vi "Obtain Request Events.vi"(8 "error in (no error)":errorcluster, 10 "Create New?":bool) -> (0 "error out":errorcluster, 2 "Tool Module Request Events":T1)   [LabVIEW 2015, in "Tool Module.lvlib"]
doc: "This VI Obtains/Creates the Requests events that will be used for other modules to communicate with the module that owns this VI. These Requests events will be accessed only via Public API methods for this module.\n\n<b>NOTE</b>: The contents of this VI are automatically generated and modified by the <b>Tools > Delacor > DQMH</b> utilities. Consider using those utilities instead of making your own modifications to this VI.\n_____\nBased on Delacor QMH Project Template 2.1.0.2."
uses:
  Tool Module.lvlib
  Request Events--cluster.ctl
  Stop Argument--cluster.ctl
  Get Module Execution Status Argument--cluster.ctl
  Show Diagram Argument--cluster.ctl
  Test Trig 2 Argument--cluster.ctl
  Support/Timer Setup Params Typedef.ctl
  GOTO Argument--cluster.ctl
  Support/_GoTo Cmd Typedef--enum.ctl
  Start Inspect Argument--cluster.ctl
  Support/_Sample Data Rtn Cluster--typedef.ctl
  CONNECT Argument--cluster.ctl
  Get All Inspect Data Argument--cluster.ctl
  Get All Inspect Data (Reply Payload)--cluster.ctl
  Get Inspection Limits Argument--cluster.ctl
  Get Inspection Limits (Reply Payload)--cluster.ctl
  Set Inspection Limits Argument--cluster.ctl
  Support/_Inspection Limits cluster--typedef.ctl
  Update Status Argument--cluster.ctl
  Start Data Monitor Argument--cluster.ctl
  Get FPGA Setup Params Argument--cluster.ctl
  Get FPGA Setup Params (Reply Payload)--cluster.ctl
  Tool Typedefs/_FPGA Setup Params Cluster--typedef.ctl
  Tool Typedefs/_FPGA Timing Constraints Cluster--typedef.ctl
  Tool Typedefs/_FPGA Timing Ctrl Cluster--typedef.ctl
  Tool Typedefs/_FPGA Laser Config Cluster--typedef.ctl
  Tool Typedefs/_FPGA Peak Proc Cfg Cluster--typedef.ctl
  Tool Typedefs/_FPGA SPI Cfg Cluster--typedef.ctl
  Set FPGA Setup Params Argument--cluster.ctl
  Set Tool Config Argument--cluster.ctl
  Tool Config/_Configuration Cluster_v3--typedef.ctl
  Tool Config/_Tool Block Cluster_v3--typedef.ctl
  Tool Config/_Motor Block Cluster_v2--typedef.ctl
  Tool Config/_Verification Blk Cluster--typedef.ctl
  Tool Config/_ProbeConfigParams Cluster--typedef.ctl
  Tool Config/_Sensor Block Cluster--typedef.ctl
  Tool Config/_SensorConfigParams Cluster--typedef.ctl
  Get Tool Config Argument--cluster.ctl
  Get Tool Config (Reply Payload)--cluster.ctl
  Set Integration Count Argument--cluster.ctl
  Set Laser Params Argument--cluster.ctl
  Get Mtrl Ctrl Reg Argument--cluster.ctl
  Get Mtrl Ctrl Reg (Reply Payload)--cluster.ctl
  Commit Ctrl Reg Argument--cluster.ctl
  Set Event Logger Argument--cluster.ctl
  Event Logger Library/Event Log/EventLog.lvclass
  Write to File Argument--cluster.ctl
  Read from File Argument--cluster.ctl
  Set Device Temp Thresholds Argument--cluster.ctl
  Tool Typedefs/_Temperature Threshold Arrays--typedef.ctl
  Get Cycle Count Argument--cluster.ctl
  Get Cycle Count (Reply Payload)--cluster.ctl
  Return FPGA Setup Data Argument--cluster.ctl
  Return FPGA Setup Data (Reply Payload)--cluster.ctl
  Update FPGA Setup Data Argument--cluster.ctl
  Tool Config/Tool Cfg.lvlib
panel:
  # "NOTE: The contents of this VI are automatically generated and modified by the Tools > Delacor > DQMH utilities. Consider using those utilities instead of making your own modifications to this VI."
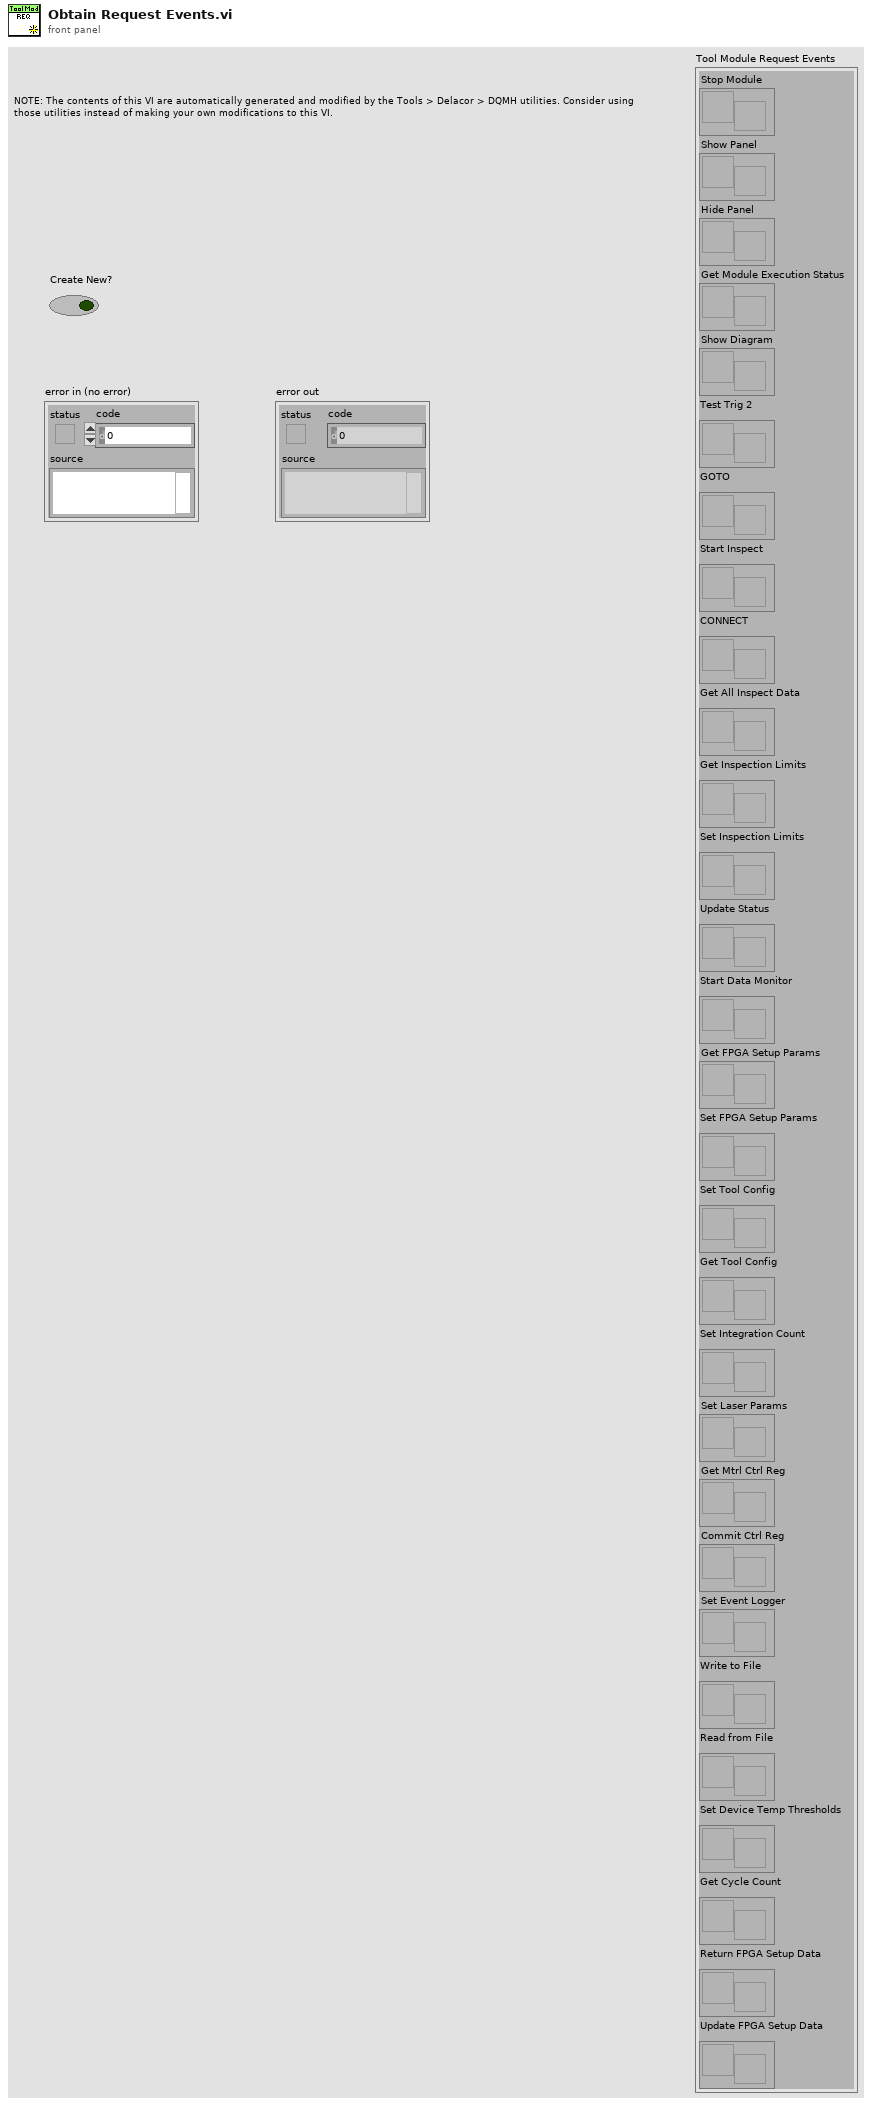
[diagram p1: front panel]
types:
  T1 = typedef "Tool Module.lvlib/Request Events--cluster.ctl" = cluster{"Stop Module":refnum<user-event>, "Show Panel":refnum<user-event>, "Hide Panel":refnum<user-event>, "Get Module Execution Status":refnum<user-event>, "Show Diagram":refnum<user-event>, "Test Trig 2":refnum<user-event>, "GOTO":refnum<user-event>, "Start Inspect":refnum<user-event>, "CONNECT":refnum<user-event>, "Get All Inspect Data":refnum<user-event>, "Get Inspection Limits":refnum<user-event>, "Set Inspection Limits":refnum<user-event>, "Update Status":refnum<user-event>, "Start Data Monitor":refnum<user-event>, "Get FPGA Setup Params":refnum<user-event>, "Set FPGA Setup Params":refnum<user-event>, "Set Tool Config":refnum<user-event>, "Get Tool Config":refnum<user-event>, "Set Integration Count":refnum<user-event>, "Set Laser Params":refnum<user-event>, "Get Mtrl Ctrl Reg":refnum<user-event>, "Commit Ctrl Reg":refnum<user-event>, "Set Event Logger":refnum<user-event>, "Write to File":refnum<user-event>, "Read from File":refnum<user-event>, "Set Device Temp Thresholds":refnum<user-event>, "Get Cycle Count":refnum<user-event>, "Return FPGA Setup Data":refnum<user-event>, "Update FPGA Setup Data":refnum<user-event>}
  T2 = typedef "Tool Module.lvlib/Update FPGA Setup Data Argument--cluster.ctl" = cluster{"Commit":bool, "FPGA Setup Parameters":T3}
  T3 = typedef "_FPGA Setup Params Cluster--typedef.ctl" = cluster{"FPGA Timing Constraints":T4, "FPGA Timing Ctrl":T5, "FPGA Laser Config":T6, "FPGA Peak Proc Cfg":T7, "FPGA SPI Cfg":T8}
  T4 = typedef "_FPGA Timing Constraints Cluster--typedef.ctl" = cluster{"frame.length Min":u16, "frame.ST_OFF Min":u16, "frame.ST_ON Min":u16, "frame.first data idx":u16, "frame.integ Offset":u16, "frame.integ Delay":u16, "frame.ad_latch Delay":u16, "frame.trig time Max":u32}
  T5 = typedef "_FPGA Timing Ctrl Cluster--typedef.ctl" = cluster{"trig.time":u32, "integ.count 1":u32, "integ.count 2":u32, "encdr.latch ctrl":u32, "pixel.read count":u16, "clock.select":u16, "ad.clock offset":u16, "data.control reg":u16}
  T6 = typedef "_FPGA Laser Config Cluster--typedef.ctl" = cluster{"laser.gain":i16, "laser.threshold Low":u16, "laser.threshold High":u16, "laser.dac init":u16, "laser.dac Min":u16, "laser.dac Max":u16, "laser.config reg":u16}
  T7 = typedef "_FPGA Peak Proc Cfg Cluster--typedef.ctl" = cluster{"PD.threshold":u16, "PD.width detect Min":u8, "PD.sensor pixels":u16, "PD.config reg":u16}
  T8 = typedef "_FPGA SPI Cfg Cluster--typedef.ctl" = cluster{"SPI Divide Value":u8, "SPI config reg":u16}
  T9 = typedef "Tool Module.lvlib/Return FPGA Setup Data Argument--cluster.ctl" = cluster{"Reload":bool, "Wait Notifier":refnum<notifier>, "wait for reply":bool}
  T10 = typedef "Tool Module.lvlib/Get Cycle Count Argument--cluster.ctl" = cluster{"Clear?":bool, "Wait Notifier":refnum<notifier>}
  T11 = typedef "Tool Module.lvlib/Set Device Temp Thresholds Argument--cluster.ctl" = cluster{"Device Temp Thold Arrays":T12}
  T12 = typedef "_Temperature Threshold Arrays--typedef.ctl" = cluster{"High Thold ":dbl[], "Low Thold ":dbl[]}
  T13 = typedef "Tool Module.lvlib/Read from File Argument--cluster.ctl" = cluster{"Filename":string, "Create?":bool, "Flattened Data Strings":string[]}
  T14 = typedef "Tool Module.lvlib/Write to File Argument--cluster.ctl" = cluster{"Filename":string, "Flattened data strings":string[]}
  T15 = typedef "Tool Module.lvlib/Set Event Logger Argument--cluster.ctl" = cluster{"EventLog.lvclass":refnum<class "EventLog.lvclass">}
  T16 = typedef "Tool Module.lvlib/Commit Ctrl Reg Argument--cluster.ctl" = cluster{"Ctrl Reg":u16}
  T17 = typedef "Tool Module.lvlib/Get Mtrl Ctrl Reg Argument--cluster.ctl" = cluster{"dummy":bool, "Wait Notifier":refnum<notifier>}
  T18 = typedef "Tool Module.lvlib/Set Laser Params Argument--cluster.ctl" = cluster{"Mode":i16, "Gain":u16, "Init DAC":u16}
  T19 = typedef "Tool Module.lvlib/Set Integration Count Argument--cluster.ctl" = cluster{"Mode":i16, "Integ Count":u32}
  T20 = typedef "Tool Module.lvlib/Get Tool Config Argument--cluster.ctl" = cluster{"dummy":bool, "Wait Notifier":refnum<notifier>}
  T21 = typedef "Tool Module.lvlib/Set Tool Config Argument--cluster.ctl" = cluster{"Commit":bool, "Tool Config Cluster":T22}
  T22 = typedef "Tool Cfg.lvlib/_Configuration Cluster_v3--typedef.ctl" = cluster{"Tool Type":u16, "Tool SN":u16, "Tool Block":T23, "Motor Block":T24, "Verification Block":T25, "Probe Block":cluster{"nProbes":u16, "Probe Param Array":T26[]}}
  T23 = typedef "Tool Cfg.lvlib/_Tool Block Cluster_v3--typedef.ctl" = cluster{"Encoder Size":u16, "Encoder Scale":u32, "Encoder Offset":i32, "MaxEncoder":i32, "MinEncoder":i32, "Start Delay":sgl, "Tool Face Ref":sgl}
  T24 = typedef "Tool Cfg.lvlib/_Motor Block Cluster_v2--typedef.ctl" = cluster{"MinMotor Speed":u16, "MaxMotor Speed":u16, "Homing Speed":u16, "Jog Speed":u16, "Inspect Speed":u16, "VBlk Speed":u16, "CleaningPos":i32, "Safe Zone":i32, "Has Motor":bool, "Use Home Index":bool}
  T25 = typedef "Tool Cfg.lvlib/_Verification Blk Cluster--typedef.ctl" = cluster{"Angle":sgl, "FlankLength1":sgl, "FlankLength2":sgl, "Location":sgl, "Serial Number":u16}
  T26 = typedef "Tool Cfg.lvlib/_ProbeConfigParams Cluster--typedef.ctl" = cluster{"Name":string, "Laser Init Pwr":u16, "Laser Gain":u8, "Integ Count":u16, "Meas. Range":sgl, "Angle":sgl, "Probe Offset":sgl, "Sensor Block":T27}
  T27 = typedef "Tool Cfg.lvlib/_Sensor Block Cluster--typedef.ctl" = cluster{"nSensors":u16, "SensorCfgParams Array":T28[]}
  T28 = typedef "Tool Cfg.lvlib/_SensorConfigParams Cluster--typedef.ctl" = cluster{"Total Pixels":u16, "Positive  Peaks":bool, "CalibrCoefArray":dbl[], "Start Idx":u16, "End Idx":u16}
  T29 = typedef "Tool Module.lvlib/Set FPGA Setup Params Argument--cluster.ctl" = cluster{"Commit":bool, "FPGA Setup Parameters":T3}
  T30 = typedef "Tool Module.lvlib/Get FPGA Setup Params Argument--cluster.ctl" = cluster{"dummy":bool, "Wait Notifier":refnum<notifier>}
  T31 = typedef "Tool Module.lvlib/Start Data Monitor Argument--cluster.ctl" = cluster{"Monitor":bool, "Lasers ON?":bool, "Host Sample Data notifier":refnum<notifier>}
  T32 = typedef "Tool Module.lvlib/Update Status Argument--cluster.ctl" = cluster{"Encoder":i32, "STATUS":u16, "MC SM State":u16, "M_Ctrl":u16}
  T33 = typedef "Tool Module.lvlib/Set Inspection Limits Argument--cluster.ctl" = cluster{"Inspection Limits":T34}
  T34 = typedef "Tool Module.lvlib/_Inspection Limits cluster--typedef.ctl" = cluster{"MaxSamples":i32, "PosToStartScan":i32, "PosToEndScan":i32, "ScanLength":i32}
  T35 = typedef "Tool Module.lvlib/Get Inspection Limits Argument--cluster.ctl" = cluster{"dummy":bool, "Wait Notifier":refnum<notifier>}
  T36 = typedef "Tool Module.lvlib/Get All Inspect Data Argument--cluster.ctl" = cluster{"dummy":bool, "Wait Notifier":refnum<notifier>}
  T37 = typedef "Tool Module.lvlib/CONNECT Argument--cluster.ctl" = cluster{"Connect":bool}
  T38 = typedef "Tool Module.lvlib/Start Inspect Argument--cluster.ctl" = cluster{"Inspect":bool, "Host Sample Data notifier":refnum<notifier>}
  T39 = typedef "Tool Module.lvlib/GOTO Argument--cluster.ctl" = cluster{"GoTo Cmd":T40, "Data":i32}
  T40 = typedef "Tool Module.lvlib/_GoTo Cmd Typedef--enum.ctl" = enum16{"MoveA", "MoveR", "Home Position", "Home None", "Cleaning Position"}
  T41 = typedef "Tool Module.lvlib/Test Trig 2 Argument--cluster.ctl" = cluster{"Trigger Params":T42}
  T42 = typedef "Tool Module.lvlib/Timer Setup Params Typedef.ctl" = cluster{"Timer On":bool, "Period":i32, "Count":i32}
  T43 = typedef "Tool Module.lvlib/Show Diagram Argument--cluster.ctl" = cluster{"Debug?":bool}
  T44 = typedef "Tool Module.lvlib/Get Module Execution Status Argument--cluster.ctl" = cluster{"Running?":bool}
  T45 = typedef "Tool Module.lvlib/Stop Argument--cluster.ctl" = cluster{"Origin":string, "Exit via Stop Module Req?":bool, "Wait for Module to stop?":bool}
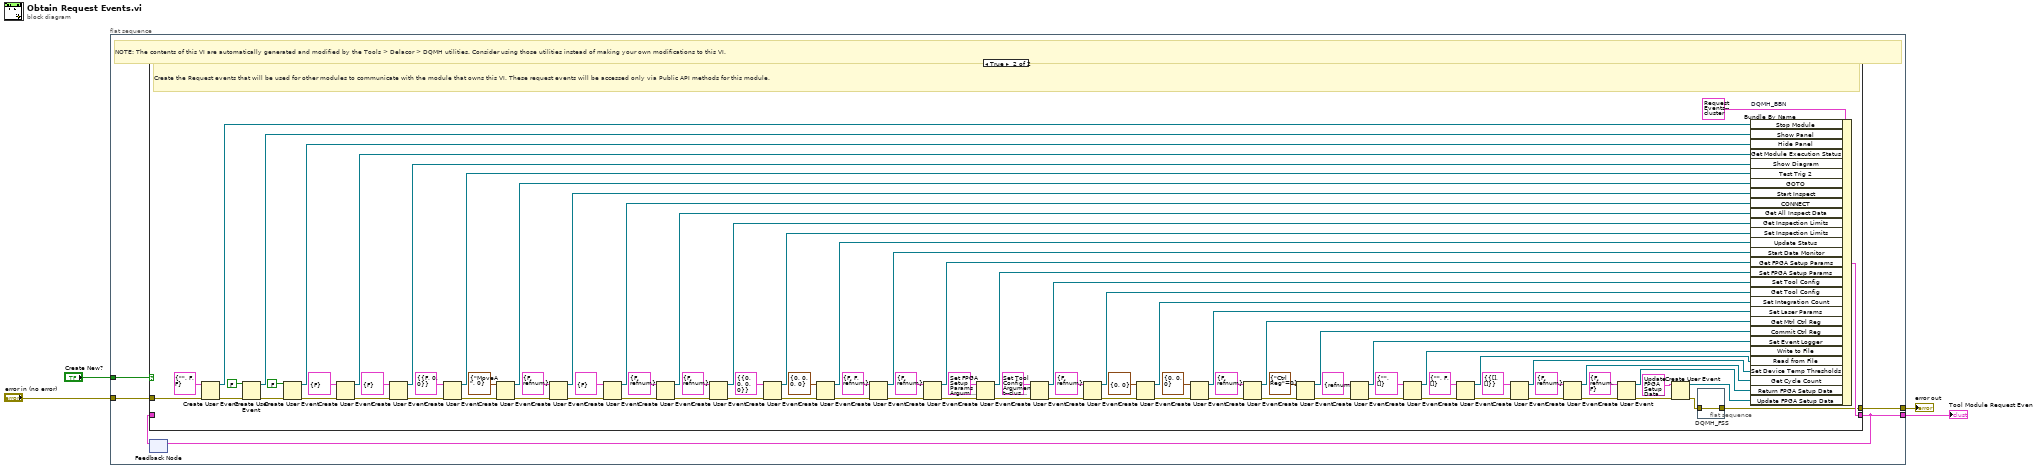
[diagram p0: block diagram]
diagram:
  n1 = flat-sequence {
    tunnel: [w9] -> w4
    tunnel: "error in (no error)" -> [w8]
    tunnel: [w6] -> w2
    tunnel: "Create New?" -> [w5]
    frame #0 {
      # "NOTE: The contents of this VI are automatically generated and modified by the Tools > Delacor > DQMH utilities. Consider using those utilities instead of making your own modifications to this VI."
      n2 = feedback #1() -> (w7:T1)  [unwired: 1 in]
      n3 = case shown="True" w5 {
        tunnel: [w10 w90] -> w9
        tunnel: w8 -> [w10 w102]
        tunnel: [w11 w99] -> w6
        tunnel: w7 -> [w11 _]
        frame False {
          # "Obtain the Request events that were created in a previous call to this VI."
        }
        frame True {
          # "Create the Request events that will be used for other modules to communicate with the module that owns this VI. These request events will be accessed only via Public API methods for this module."
          n4 = Create User Event(user event datatype=T45 {"Origin"="", "Exit via Stop Module Req?"=FALSE, "Wait for Module to stop?"=FALSE} ("Stop Argument"), error in=w102) -> (user event=w100:refnum<user-event>, error out=w97:errorcluster)
          n5 = Create User Event(user event datatype=FALSE ("Show Panel"), error in=w97) -> (user event=w95:refnum<user-event>, error out=w93:errorcluster)
          n6 = Create User Event(user event datatype=FALSE ("Hide Panel"), error in=w93) -> (user event=w92:refnum<user-event>, error out=w91:errorcluster)
          n7 = Create User Event(user event datatype=T44 {"Running?"=FALSE} ("Get Module Execution Status Argument"), error in=w91) -> (user event=w88:refnum<user-event>, error out=w89:errorcluster)
          n8 = Create User Event(user event datatype=T43 {"Debug?"=FALSE} ("Show Diagram Argument"), error in=w89) -> (user event=w85:refnum<user-event>, error out=w86:errorcluster)
          n9 = Create User Event(user event datatype=T41 {"Trigger Params"={"Timer On"=FALSE, "Period"=0, "Count"=0}} ("Test Trig 2 Argument"), error in=w86) -> (user event=w82:refnum<user-event>, error out=w83:errorcluster)
          n10 = Create User Event(user event datatype=T39 {"GoTo Cmd"=enum."MoveA", "Data"=0} ("GOTO Argument"), error in=w83) -> (user event=w79:refnum<user-event>, error out=w80:errorcluster)
          n11 = Create User Event(user event datatype=T38 {"Inspect"=FALSE, "Host Sample Data notifier"=refnum} ("Start Inspect Argument"), error in=w80) -> (user event=w76:refnum<user-event>, error out=w77:errorcluster)
          n12 = Create User Event(user event datatype=T37 {"Connect"=FALSE} ("CONNECT Argument"), error in=w77) -> (user event=w73:refnum<user-event>, error out=w74:errorcluster)
          n13 = Create User Event(user event datatype=T36 {"dummy"=FALSE, "Wait Notifier"=refnum} ("Get All Inspect Data Argument"), error in=w74) -> (user event=w70:refnum<user-event>, error out=w71:errorcluster)
          n14 = Create User Event(user event datatype=T35 {"dummy"=FALSE, "Wait Notifier"=refnum} ("Get Inspection Limits Argument"), error in=w71) -> (user event=w67:refnum<user-event>, error out=w68:errorcluster)
          n15 = Create User Event(user event datatype=T33 {"Inspection Limits"={"MaxSamples"=0, "PosToStartScan"=0, "PosToEndScan"=0, "ScanLength"=0}} ("Set Inspection Limits Argument"), error in=w68) -> (user event=w64:refnum<user-event>, error out=w65:errorcluster)
          n16 = Create User Event(user event datatype=T32 {"Encoder"=0, "STATUS"=0, "MC SM State"=0, "M_Ctrl"=0} ("Update Status Argument"), error in=w65) -> (user event=w61:refnum<user-event>, error out=w62:errorcluster)
          n17 = Create User Event(user event datatype=T31 {"Monitor"=FALSE, "Lasers ON?"=FALSE, "Host Sample Data notifier"=refnum} ("Start Data Monitor Argument"), error in=w62) -> (user event=w58:refnum<user-event>, error out=w59:errorcluster)
          n18 = Create User Event(user event datatype=T30 {"dummy"=FALSE, "Wait Notifier"=refnum} ("Get FPGA Setup Params Argument"), error in=w59) -> (user event=w55:refnum<user-event>, error out=w56:errorcluster)
          n19 = Create User Event(user event datatype=T29 {"Commit"=FALSE, "FPGA Setup Parameters"={"FPGA Timing Constraints"={"frame.length Min"=530, "frame.ST_OFF Min"=15, "frame.ST_ON Min"=8, "frame.first data idx"=14, "frame.integ Offset"=6, "frame.integ Delay"=3, "frame.ad_latch Delay"=11, "frame.trig time Max"=0}, "FPGA Timing Ctrl"={"trig.time"=220, "integ.count 1"=400, "integ.count 2"=350, "encdr.latch ctrl"=1, "pixel.read count"=512, "clock.select"=2, "ad.clock offset"=16, "data.control reg"=2}, "FPGA Laser Config"={"laser.gain"=10, "laser.threshold Low"=1400, "laser.threshold High"=1900, "laser.dac init"=912, "laser.dac Min"=800, "laser.dac Max"=4000, "laser.config reg"=3}, "FPGA Peak Proc Cfg"={"PD.threshold"=0, "PD.width detect Min"=0, "PD.sensor pixels"=512, "PD.config reg"=23}, "FPGA SPI Cfg"={"SPI Divide Value"=1, "SPI config reg"=1}}} ("Set Cur FPGA Setup Params Argument"), error in=w56) -> (user event=w52:refnum<user-event>, error out=w53:errorcluster)
          n20 = Create User Event(user event datatype=T21 {"Commit"=FALSE, "Tool Config Cluster"={"Tool Type"=0, "Tool SN"=0, "Tool Block"={"Encoder Size"=0, "Encoder Scale"=0, "Encoder Offset"=0, "MaxEncoder"=0, "MinEncoder"=0, "Start Delay"=0.0, "Tool Face Ref"=0.0}, "Motor Block"={"MinMotor Speed"=0, "MaxMotor Speed"=0, "Homing Speed"=90, "Jog Speed"=90, "Inspect Speed"=90, "VBlk Speed"=90, "CleaningPos"=0, "Safe Zone"=0, "Has Motor"=FALSE, "Use Home Index"=FALSE}, "Verification Block"={"Angle"=90.0, "FlankLength1"=0.0, "FlankLength2"=0.0, "Location"=0.0, "Serial Number"=0}, "Probe Block"={"nProbes"=0, "Probe Param Array"=[]}}} ("Set Tool Config Argument"), error in=w53) -> (user event=w49:refnum<user-event>, error out=w50:errorcluster)
          n21 = Create User Event(user event datatype=T20 {"dummy"=FALSE, "Wait Notifier"=refnum} ("Get Tool Config Argument"), error in=w50) -> (user event=w46:refnum<user-event>, error out=w47:errorcluster)
          n22 = Create User Event(user event datatype=T19 {"Mode"=0, "Integ Count"=0} ("Set Integration Count Argument"), error in=w47) -> (user event=w43:refnum<user-event>, error out=w44:errorcluster)
          n23 = Create User Event(user event datatype=T18 {"Mode"=0, "Gain"=0, "Init DAC"=0} ("Set Laser Params Argument"), error in=w44) -> (user event=w40:refnum<user-event>, error out=w41:errorcluster)
          n24 = Create User Event(user event datatype=T17 {"dummy"=FALSE, "Wait Notifier"=refnum} ("Get Mtrl Ctrl Reg Argument"), error in=w41) -> (user event=w37:refnum<user-event>, error out=w38:errorcluster)
          n25 = Create User Event(user event datatype=T16 {"Ctrl Reg"=0} ("Set Mtr Ctrl Reg Argument"), error in=w38) -> (user event=w34:refnum<user-event>, error out=w35:errorcluster)
          n26 = Create User Event(user event datatype=T15 {"EventLog.lvclass"=refnum} ("Set Event Logger Argument"), error in=w35) -> (user event=w31:refnum<user-event>, error out=w32:errorcluster)
          n27 = Create User Event(user event datatype=T14 {"Filename"="", "Flattened data strings"=[]} ("Write to File Argument"), error in=w32) -> (user event=w28:refnum<user-event>, error out=w29:errorcluster)
          n28 = Create User Event(user event datatype=T13 {"Filename"="", "Create?"=FALSE, "Flattened Data Strings"=[]} ("Read from File Argument"), error in=w29) -> (user event=w25:refnum<user-event>, error out=w26:errorcluster)
          n29 = Create User Event(user event datatype=T11 {"Device Temp Thold Arrays"={"High Thold "=[], "Low Thold "=[]}} ("Set Device Temp Thresholds Argument"), error in=w26) -> (user event=w22:refnum<user-event>, error out=w23:errorcluster)
          n30 = Create User Event(user event datatype=T10 {"Clear?"=FALSE, "Wait Notifier"=refnum} ("Get Cycle Count Argument"), error in=w23) -> (user event=w19:refnum<user-event>, error out=w20:errorcluster)
          n31 = Create User Event(user event datatype=T9 {"Reload"=FALSE, "Wait Notifier"=refnum, "wait for reply"=FALSE} ("Return FPGA Setup Data Argument"), error in=w20) -> (user event=w16:refnum<user-event>, error out=w17:errorcluster)
          n32 = Create User Event(user event datatype=T2 {"Commit"=FALSE, "FPGA Setup Parameters"={"FPGA Timing Constraints"={"frame.length Min"=530, "frame.ST_OFF Min"=15, "frame.ST_ON Min"=8, "frame.first data idx"=14, "frame.integ Offset"=6, "frame.integ Delay"=3, "frame.ad_latch Delay"=11, "frame.trig time Max"=0}, "FPGA Timing Ctrl"={"trig.time"=220, "integ.count 1"=400, "integ.count 2"=350, "encdr.latch ctrl"=1, "pixel.read count"=512, "clock.select"=2, "ad.clock offset"=16, "data.control reg"=2}, "FPGA Laser Config"={"laser.gain"=10, "laser.threshold Low"=1400, "laser.threshold High"=1900, "laser.dac init"=912, "laser.dac Min"=800, "laser.dac Max"=4000, "laser.config reg"=3}, "FPGA Peak Proc Cfg"={"PD.threshold"=0, "PD.width detect Min"=0, "PD.sensor pixels"=512, "PD.config reg"=23}, "FPGA SPI Cfg"={"SPI Divide Value"=1, "SPI config reg"=1}}} ("Update FPGA Setup Data Argument"), error in=w17) -> (user event=w13:refnum<user-event>, error out=w14:errorcluster)
          n33 = flat-sequence "DQMH_FSS" {
            tunnel: w14 -> [w103]
            tunnel: [w103] -> w90
            frame #0 {
            }
          }
          n34 = Bundle By Name "DQMH_BBN"(cluster=T1 {"Stop Module"=refnum, "Show Panel"=refnum, "Hide Panel"=refnum, "Get Module Execution Status"=refnum, "Show Diagram"=refnum, "Test Trig 2"=refnum, "GOTO"=refnum, "Start Inspect"=refnum, "CONNECT"=refnum, "Get All Inspect Data"=refnum, "Get Inspection Limits"=refnum, "Set Inspection Limits"=refnum, "Update Status"=refnum, "Start Data Monitor"=refnum, "Get FPGA Setup Params"=refnum, "Set FPGA Setup Params"=refnum, "Set Tool Config"=refnum, "Get Tool Config"=refnum, "Set Integration Count"=refnum, "Set Laser Params"=refnum, "Get Mtrl Ctrl Reg"=refnum, "Commit Ctrl Reg"=refnum, "Set Event Logger"=refnum, "Write to File"=refnum, "Read from File"=refnum, "Set Device Temp Thresholds"=refnum, "Get Cycle Count"=refnum, "Return FPGA Setup Data"=refnum, "Update FPGA Setup Data"=refnum} ("output cluster"), "Stop Module"=w100, "Show Panel"=w95, "Hide Panel"=w92, "Get Module Execution Status"=w88, "Show Diagram"=w85, "Test Trig 2"=w82, "GOTO"=w79, "Start Inspect"=w76, "CONNECT"=w73, "Get All Inspect Data"=w70, "Get Inspection Limits"=w67, "Set Inspection Limits"=w64, "Update Status"=w61, "Start Data Monitor"=w58, "Get FPGA Setup Params"=w55, "Set FPGA Setup Params"=w52, "Set Tool Config"=w49, "Get Tool Config"=w46, "Set Integration Count"=w43, "Set Laser Params"=w40, "Get Mtrl Ctrl Reg"=w37, "Commit Ctrl Reg"=w34, "Set Event Logger"=w31, "Write to File"=w28, "Read from File"=w25, "Set Device Temp Thresholds"=w22, "Get Cycle Count"=w19, "Return FPGA Setup Data"=w16, "Update FPGA Setup Data"=w13) -> (w99:T1)
        }
      }
      n35 = feedback-in #1(w6) -> ()
    }
  }
  "Tool Module Request Events" <- w2
  "error out" <- w4
